vi "Untitled 3.vi"() -> ()   [LabVIEW 2014]
uses:
  <vilib>/Utility/miscctls.llb/LVDateTimeRec.ctl
panel:
  out "date time rec":T1
  out "date/time string 2":string
  out "date/time string":string
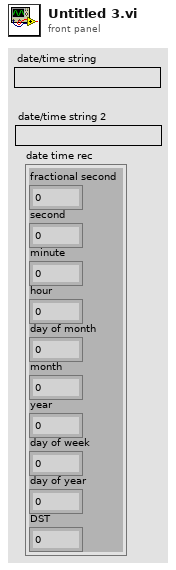
[diagram p1: front panel]
types:
  T1 = typedef "LVDateTimeRec.ctl" = cluster{"fractional second":dbl, "second":i32, "minute":i32, "hour":i32, "day of month":i32, "month":i32, "year":i32, "day of week":i32, "day of year":i32, "DST":i32}
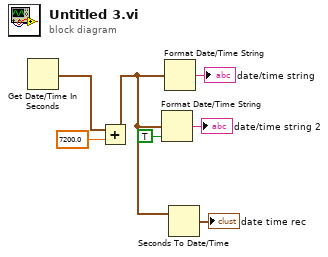
[diagram p0: block diagram]
diagram:
  n1 = Get Date/Time In Seconds() -> (seconds since 1Jan1904=w2:timestamp)
  n2 = Add(x=w2, y=7200.0) -> (x+y=w1:timestamp)
  n3 = Format Date/Time String(seconds (now)=w1, UTC format=TRUE) -> (date/time string=→"date/time string 2":string)  [unwired: 1 in]
  n4 = Format Date/Time String(seconds (now)=w1) -> (date/time string=→"date/time string":string)  [unwired: 2 in]
  n5 = Seconds To Date/Time(time stamp (now)=w1) -> (date time rec=→"date time rec":T1)  [unwired: 1 in]
